vi "MVi-FW Template.vi"(8 "EorIn":errorcluster, 11 "ImgIn":T1(plugin-control)) -> (0 "ErrOut":errorcluster, 3 "ImgOut":T1(plugin-control))   [LabVIEW 2014]
doc: "Use this template to build a VI to use as a subVI."
panel:
  # "Output Parameters"
  # "Input Parameters"
  # "VI Description:\nThis VI is .."
  # ":: MVi Framework V1.0 ::\nAuthor:Gaoke Yang\nEmail: gaoke.yang@yahoo.com\nWeb: www.mvicontrol.com\nCopyright (C) 2015, MVI Technologies All Rights Reserved"
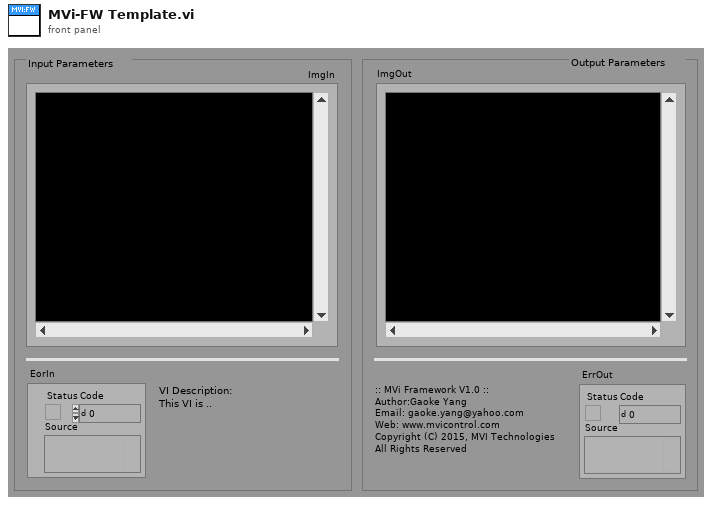
[diagram p1: front panel]
types:
  T1 = typedef "IMAQ Image.ctl" = refnum<image>
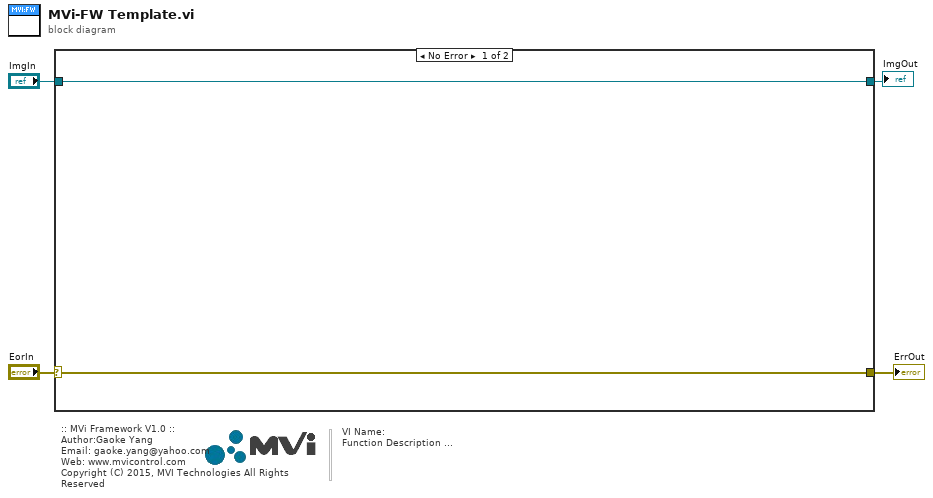
[diagram p0: block diagram]
diagram:
  # "VI Name:\nFunction Description ..."
  # ":: MVi Framework V1.0 ::\nAuthor:Gaoke Yang\nEmail: gaoke.yang@yahoo.com\nWeb: www.mvicontrol.com\nCopyright (C) 2015, MVI Technologies All Rights Reserved"
  n1 = case shown="No Error" "EorIn" {
    selector: "EorIn" -> [w6 w8]
    tunnel: [w6 w8] -> w3
    tunnel: [w5 w7] -> w1
    tunnel: "ImgIn" -> [w5 w7]
    frame No Error {
    }
    frame Error {
    }
  }
  "ErrOut" <- w3
  "ImgOut" <- w1
